vi "StateSpaceUtil_MakeWhiteNoiseVector.vi"(11 "StdDevs":T1) -> (0 "Size Coerced":bool, 3 "WhiteNoise":T1)   [LabVIEW 2019, in "Trajectory_Library.lvlib"]
doc: "Creates a vector of normally distributed white noise with the given noise intensities for each element.\n\n\nInputs:\n - stdDevs -- A matrix whose elements are the standard deviations of each element of the noise vector.\n\nOutputs:\n - WhiteNoise -- White noise vector.\n - sizeCoerced -- If TRUE, an error occured."
uses:
  Trajectory_Library.lvlib
  <vilib>/Analysis/Matrix/Datatypes/RealMatrix.ctl
  <vilib>/Analysis/NI_AALBase.lvlib
  <vilib>/Analysis/Matrix/NI_Matrix.lvlib
panel:
  # "<J ,1>"
  # "<J ,1>"
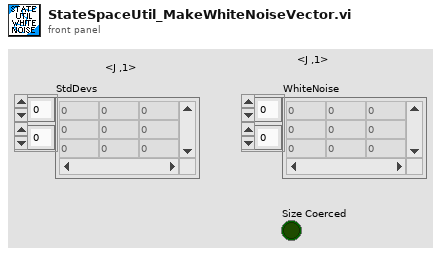
[diagram p1: front panel]
types:
  T1 = typedef "NI_Matrix.lvlib/RealMatrix.ctl" = dbl[][]
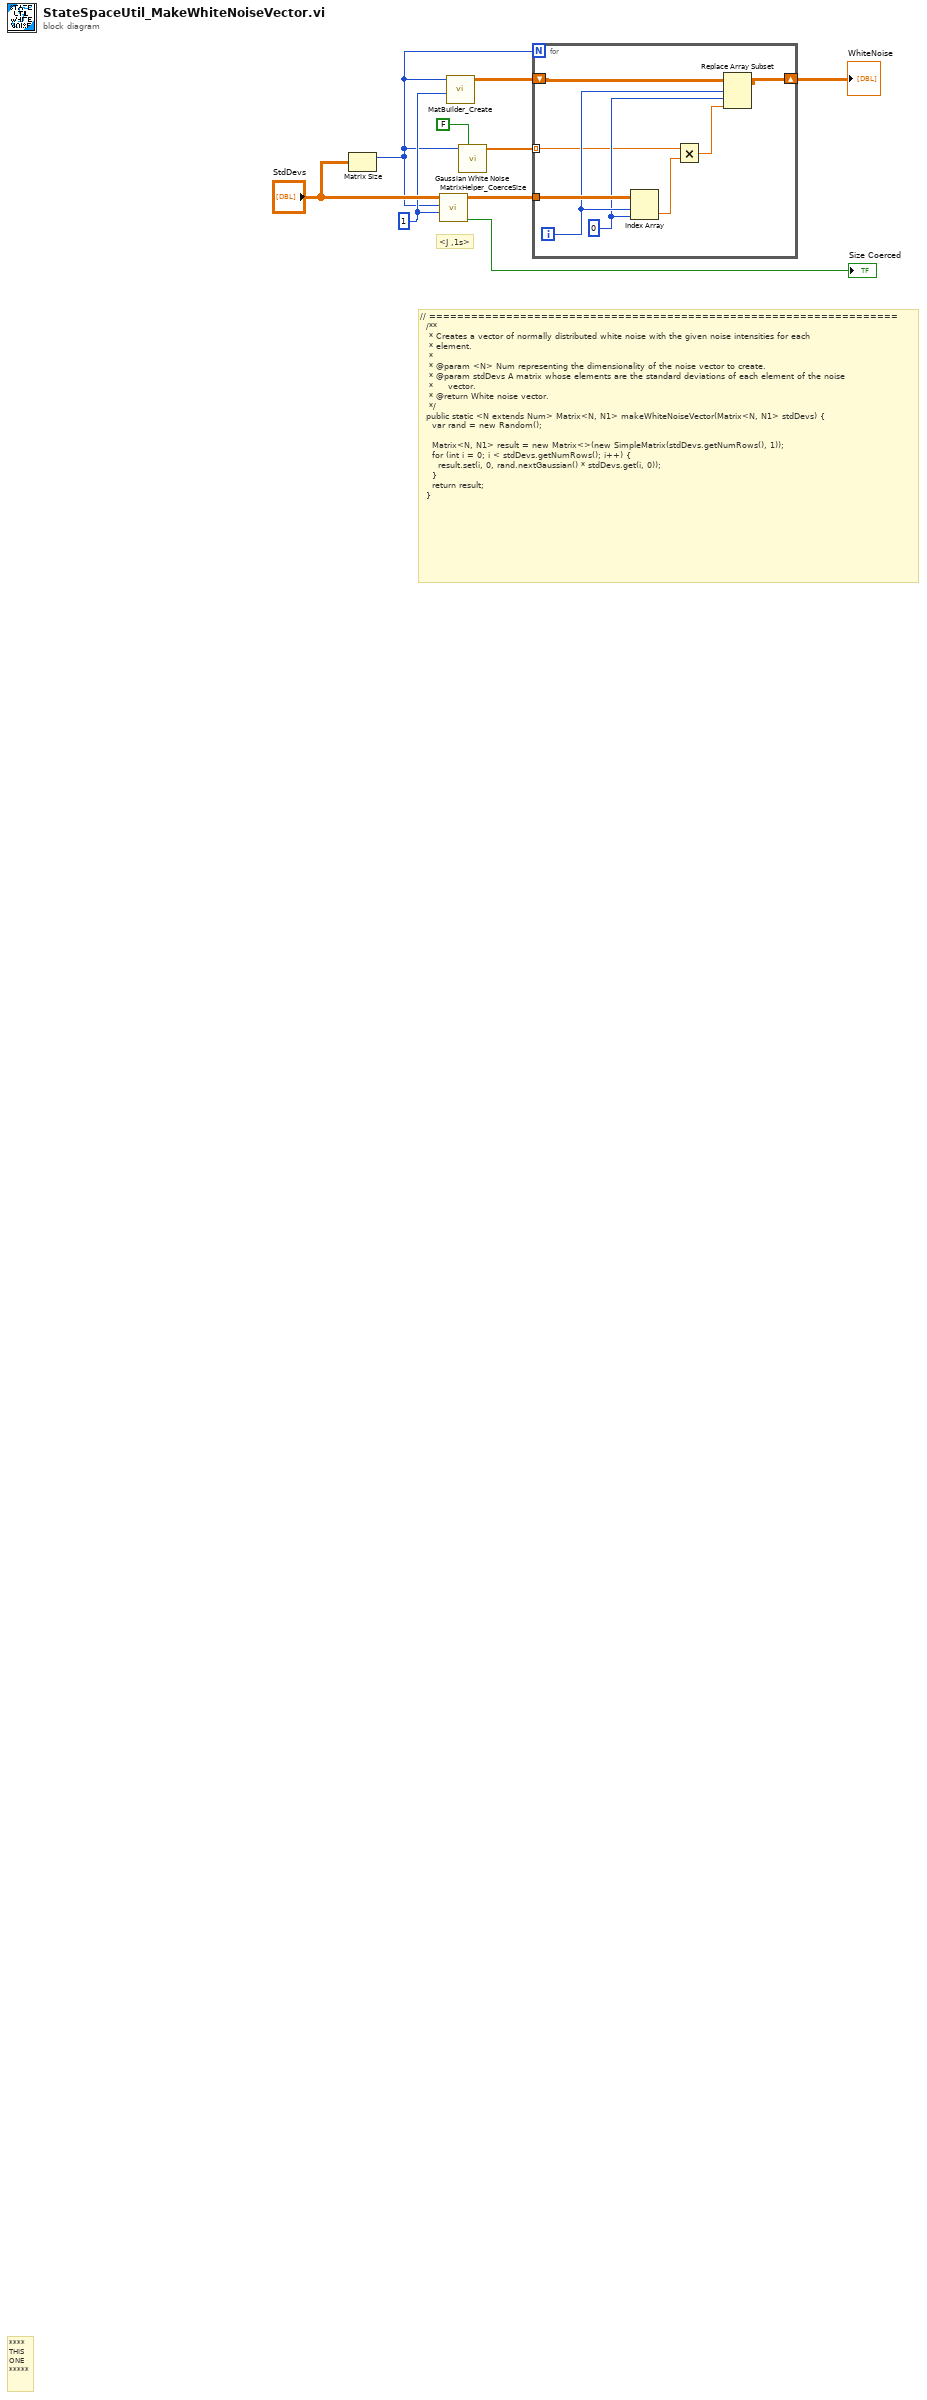
[diagram p0: block diagram]
diagram:
  w8 = 1 ("number of columns")
  # "// ===================================================================\n  /**\n   * Creates a vector of normally distributed white noise with the given noise intensities for each\n   * element.\n   *\n   * @param <N> Num representing the dimensionality of the noise vector to create.\n   * @param stdDevs A matrix whose elements are the standard deviations of each element of the noise\n   *     vector.\n   * @return White noise vector.\n   */\n  public static <N extends Num> Matrix<N, N1> makeWhiteNoiseVector(Matrix<N, N1> stdDevs) {\n    var rand = new Random();\n\n    Matrix<N, N1> result = new Matrix<>(new SimpleMatrix(stdDevs.getNumRows(), 1));\n    for (int i = 0; i < stdDevs.getNumRows(); i++) {\n      result.set(i, 0, rand.nextGaussian() * stdDevs.get(i, 0));\n    }\n    return result;\n  }"
  # "<J ,1s>"
  # "****\nTHIS\nONE\n*****"
  n1 = Matrix Size(0:"StdDevs") -> (1:w4:i32)  [unwired: 1 out]
  n2 = call "MatrixHelper_CoerceSize.vi"("Columns"=w8, "Rows"=w4, "input matrix"="StdDevs") -> ("Coerced"=→"Size Coerced":bool, "output matrix"=w3:T1)  [unwired: 7 in]
  n3 = call "MatBuilder_Create.vi"("Columns"=w8, "Rows"=w4) -> ("output matrix"=w5:T1)  [unwired: 9 in]
  n4 = call <vilib>:"Gaussian White Noise.vi"("initialize?"=FALSE, "samples"=w4) -> ("Gaussian noise pattern"=w6:dbl[])  [unwired: 8 in, 1 out]
  n5 = for {
    N: w4 -> [_]
    tunnel: w6 -> [w11] mode=indexing
    shift-right: [w14] -> w2
    shift-left: w5 -> [w15]
    tunnel: w3 -> [w17]
    i -> [w13]
    w12 = 0 ("index (col)")
    n6 = Index Array(array=w17, index (row)=w13, index (col)=w12) -> (element=w16:dbl)
    n7 = Multiply(x=w11, y=w16) -> (x*y=w10:dbl)
    n8 = Replace Array Subset(array=w15, new element=w10, index (row)=w13, index (col)=w12) -> (w14:T1)
  }
  "WhiteNoise" <- w2
